vi "Quiz3_TP059851_Sim Yoke Shin_Client.vi"() -> ()   [LabVIEW 2020]
panel:
  in  "Tab Control":enum32{"Page 1", "Page 2"}(tab)
  in  "Send to Server":bool
  in  "Y":dbl
  in  "X":dbl
  out "Devide by Zero":bool
  out "X + Y":dbl
  out "X - Y":dbl
  out "X x Y":dbl
  out "X / Y":dbl
  # "Client"
  # "Result"
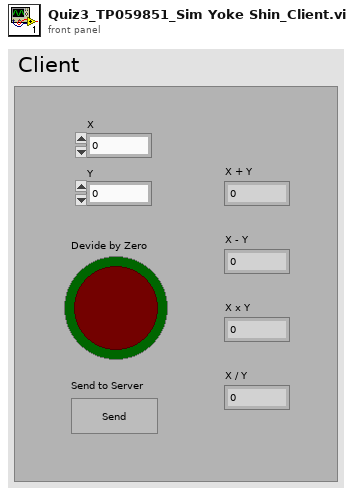
[diagram p1: front panel]
types:
  T1 = enum8{"Enabled", "Disabled", "Disabled and Grayed Out"}
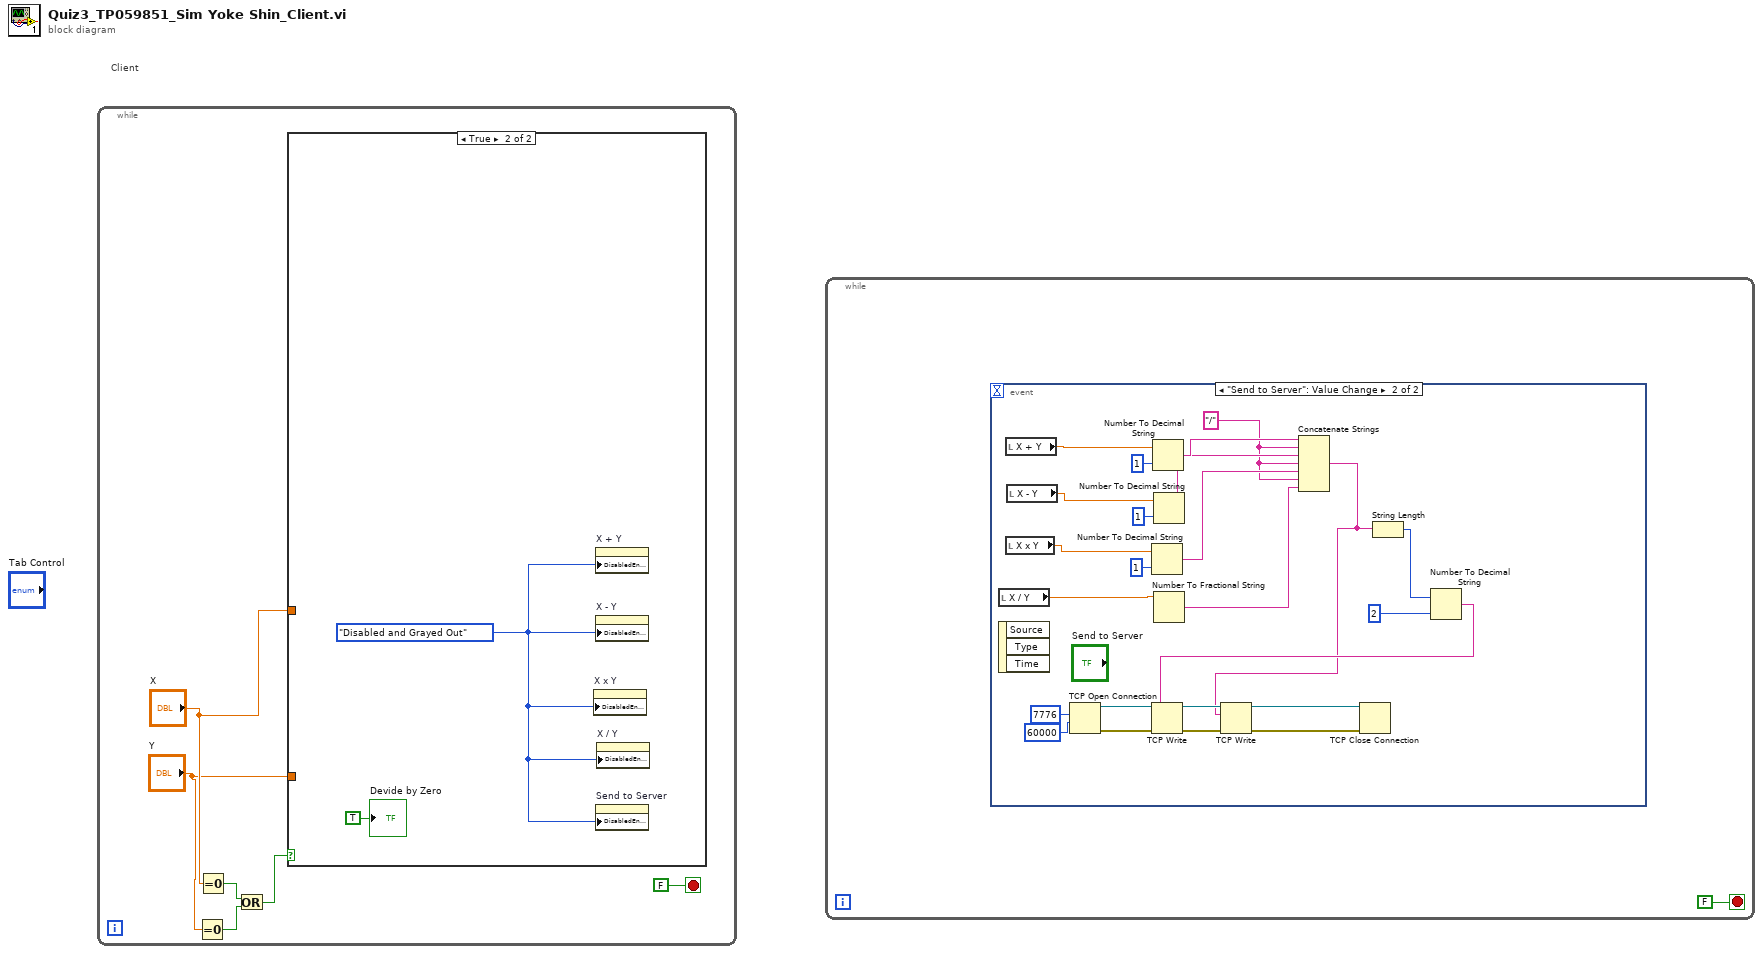
[diagram p0: block diagram]
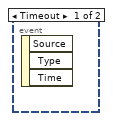
[diagram p2: hidden frame]
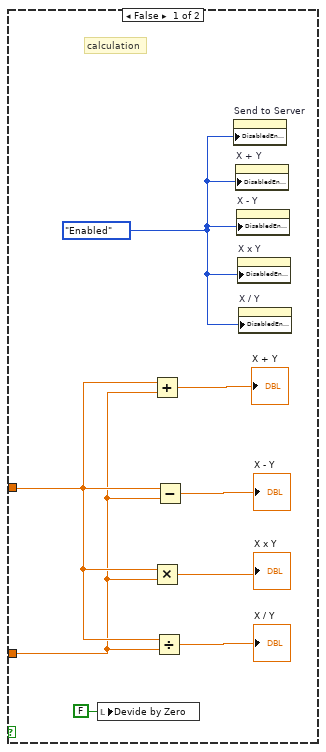
[diagram p3: hidden frame]
diagram:
  # "Client"
  n1 = while {
    stop <- FALSE stop-if-true
    n2 = Equal To 0?(x="Y") -> (x = 0?=w4:bool)
    n3 = Equal To 0?(x="X") -> (x = 0?=w5:bool)
    n4 = Or(x=w5, y=w4) -> (x .or. y?=w3:bool)
    n5 = case shown="True" w3 {
      tunnel: "X" -> [w14 _]
      tunnel: "Y" -> [w13 _]
      frame False {
        w12 = T1."Enabled" ("Disabled")
        # "calculation"
        n6 = local write "Devide by Zero"(FALSE ("Devide by Zero")) -> ()
        n7 = Add(x=w14, y=w13) -> (x+y=→"X + Y":dbl)
        n8 = Multiply(x=w14, y=w13) -> (x*y=→"X x Y":dbl)
        n9 = Divide(x=w14, y=w13) -> (x/y=→"X / Y":dbl)
        n10 = Subtract(x=w14, y=w13) -> (x-y=→"X - Y":dbl)
        n11 = property on="Send to Server" class="Bool"("DisabledEnum"=w12) -> ()  [unwired: 2 in, 2 out]
        n12 = property on="X + Y" class="DigNum (strict)"("DisabledEnum"=w12) -> ()  [unwired: 2 in, 2 out]
        n13 = property on="X - Y" class="DigNum (strict)"("DisabledEnum"=w12) -> ()  [unwired: 2 in, 2 out]
        n14 = property on="X x Y" class="DigNum (strict)"("DisabledEnum"=w12) -> ()  [unwired: 2 in, 2 out]
        n15 = property on="X / Y" class="DigNum (strict)"("DisabledEnum"=w12) -> ()  [unwired: 2 in, 2 out]
      }
      frame True {
        w16 = T1."Disabled and Grayed Out" ("Disabled")
        n16 = property on="X x Y" class="DigNum (strict)"("DisabledEnum"=w16) -> ()  [unwired: 2 in, 2 out]
        n17 = property on="X + Y" class="DigNum (strict)"("DisabledEnum"=w16) -> ()  [unwired: 2 in, 2 out]
        n18 = property on="X - Y" class="DigNum (strict)"("DisabledEnum"=w16) -> ()  [unwired: 2 in, 2 out]
        n19 = property on="Send to Server" class="Bool"("DisabledEnum"=w16) -> ()  [unwired: 2 in, 2 out]
        n20 = property on="X / Y" class="DigNum (strict)"("DisabledEnum"=w16) -> ()  [unwired: 2 in, 2 out]
        "Devide by Zero" <- TRUE ("Devide by Zero")
      }
    }
  }
  n21 = while {
    stop <- FALSE stop-if-true
    n22 = event shown="[1] \"Send to Server\": Value Change" {
      selector: _ -> [_ _]
      dyn-events: _ -> [_ _]
      timeout: _ -> [_ _]
      event Timeout {
        n23 = event-data() -> ()  [unwired: 1 in, 3 out]
      }
      event "Send to Server": Value Change {
        w21 = "/" ("string")
        n24 = local read "X / Y"() -> (w23:dbl)
        n25 = event-data() -> ()  [unwired: 1 in, 3 out]
        n26 = local read "X + Y"() -> (w32:dbl)
        n27 = local read "X x Y"() -> (w28:dbl)
        n28 = local read "X - Y"() -> (w27:dbl)
        n29 = TCP Open Connection(remote port or service name=u16 7776, timeout ms (60000)=60000) -> (connection ID=w41:refnum<k5>, error out=w20:errorcluster)  [unwired: 3 in]
        n30 = Number To Decimal String(number=w28, width (-)=i16 1) -> (decimal integer string=w24:string)
        n31 = Number To Decimal String(number=w32, width (-)=i16 1) -> (decimal integer string=w26:string)
        n32 = Number To Decimal String(number=w27, width (-)=i16 1) -> (decimal integer string=w25:string)
        n33 = Number To Fractional String(number=w23) -> (F-format string=w22:string)  [unwired: 3 in]
        n34 = Concatenate Strings(w26, w21, w25, w21, w24, w21, w22) -> (w38:string)
        n35 = String Length(string=w38) -> (length=w36:i32)
        n36 = Number To Decimal String(number=w36, width (-)=i16 2) -> (decimal integer string=w39:string)
        n37 = TCP Write(connection ID=w41, data in=w39, error in (no error)=w20) -> (connection ID out=w40:refnum<k5>, error out=w19:errorcluster)  [unwired: 1 in, 1 out]
        n38 = TCP Write(connection ID=w40, data in=w38, error in (no error)=w19) -> (connection ID out=w37:refnum<k5>, error out=w18:errorcluster)  [unwired: 1 in, 1 out]
        n39 = TCP Close Connection(connection ID=w37, error in (no error)=w18) -> ()  [unwired: 1 in, 2 out]
      }
    }
  }
